vi "Read configuration.vi"(7 "force loading?":bool=TRUE, 8 "error in (no error)":errorcluster, 11 "DAQMH121119OrcaFlash in":refnum<class "DAQOrcaFlash.lvclass">) -> (0 "error out":errorcluster, 3 "DAQMH121119OrcaFlash out":refnum<class "DAQOrcaFlash.lvclass">)   [LabVIEW 2012, in "DAQOrcaFlash.lvclass"]
doc: "Reads the XML-based configuration file and populates the configuration cluster accordingly. Configuration file name is <component ID>.xml."
uses:
  DAQOrcaFlash.lvclass
  <vilib>/Distrio/Murmex/Murmex/Murmex.lvclass
  DAQOrcaFlash.lvclass/DAQOrcaFlash.ctl
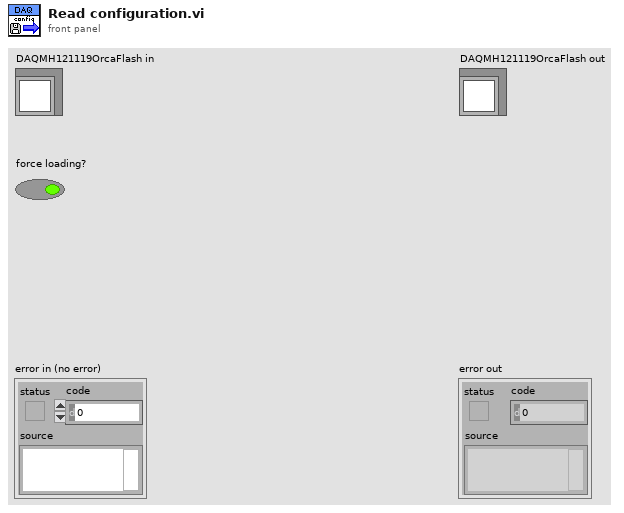
[diagram p1: front panel]
types:
  T1 = typedef "DAQOrcaFlash.lvclass/configuration_cluster.ctl" = cluster{"filepath":path, "Trigger source":T2, "Trigger mode":T3, "Sensor mode":T4, "Read out direction":T5, "Output trigger type":T6, "Output trigger source":T7, "Output trigger period":sgl[unit], "start_stop_targets":string[], "Output trigger connector":T8, "Stack component":string, "Tomo component":string, "auxiliary folder path":path, "wait before acquisition":dbl[unit], "maximum window size":i32}
  T2 = typedef "DAQOrcaFlash.lvclass/trigger_source.ctl" = sgl
  T3 = typedef "DAQOrcaFlash.lvclass/trigger_mode.ctl" = sgl
  T4 = typedef "DAQOrcaFlash.lvclass/sensor_mode.ctl" = sgl
  T5 = typedef "DAQOrcaFlash.lvclass/read out direction.ctl" = sgl
  T6 = typedef "DAQOrcaFlash.lvclass/output trigger type.ctl" = sgl
  T7 = typedef "DAQOrcaFlash.lvclass/output trigger source.ctl" = sgl
  T8 = typedef "DAQOrcaFlash.lvclass/connector.ctl" = enum32{"1", "2", "3"}
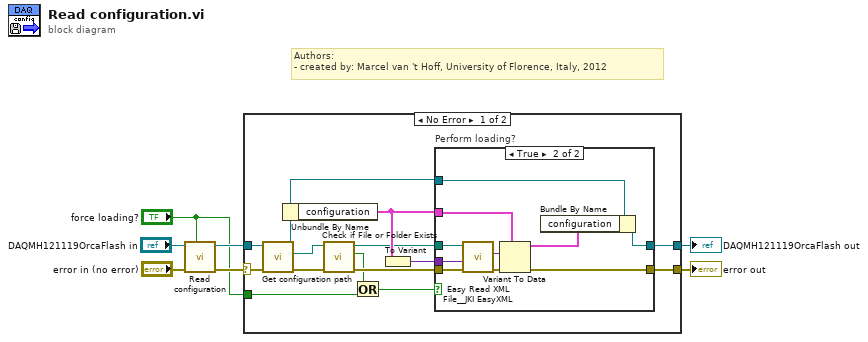
[diagram p0: block diagram]
diagram:
  # "Authors: \n- created by: Marcel van 't Hoff, University of Florence, Italy, 2012"
  n1 = call-parent "Read configuration.vi"("force loading?"="force loading?", "error in (no error)"="error in (no error)", "Murmex in"="DAQMH121119OrcaFlash in") -> ("error out"=w4:errorcluster, "Murmex out"=w5:refnum<class "DAQOrcaFlash.lvclass">)  [unwired: 7 in]
  n2 = case shown="No Error" w4 {
    selector: w4 -> [w10 w35]
    tunnel: [w18 w35] -> w1
    tunnel: [w21 w34] -> w2
    tunnel: w5 -> [w8 w34]
    tunnel: "force loading?" -> [w17 _]
    frame No Error {
      n3 = call <vilib>:"Get configuration path.vi"("error in (no error)"=w10, "Murmex in"=w8) -> ("error out"=w13:errorcluster, "configuration path"=w15:path, "Murmex out"=w9:refnum<class "DAQOrcaFlash.lvclass">)  [unwired: 7 in]
      n4 = Unbundle By Name(w9) -> ("configuration"=w19:T1)
      n5 = call <vilib>:"Check if File or Folder Exists.vi"("error in (no error)"=w13, "path"=w15) -> ("error out"=w12:errorcluster, "file or folder exists?"=w11:bool, "dup path"=w14:path)  [unwired: 7 in]
      n6 = Or(x=w11, y=w17) -> (x .or. y?=w16:bool)
      n7 = To Variant(anything=w19) -> (Variant=w20:variant)
      n8 = case "Perform loading?" shown="True" w16 {
        tunnel: [w23 w25] -> w21
        tunnel: w20 -> [_ w32]
        tunnel: w19 -> [_ w31]
        tunnel: [w22 w24] -> w18
        tunnel: w14 -> [_ w29]
        tunnel: w12 -> [w22 w28]
        tunnel: w9 -> [w23 w27]
        frame False {
        }
        frame True {
          n9 = call <vilib>:"Easy Read XML File__JKI EasyXML.vi"("error in (no error)"=w28, "LabVIEW Data (Type)"=w32, "XML File Path"=w29) -> ("error out"=w30:errorcluster, "LabVIEW Data"=w33:variant)  [unwired: 6 in, 1 out]
          n10 = Variant To Data(error in=w30, type=w31, Variant=w33) -> (data=w26:T1, error out=w24:errorcluster)
          n11 = Bundle By Name(cluster=w27, "configuration"=w26) -> (w25:refnum<class "DAQOrcaFlash.lvclass">)
        }
      }
    }
    frame Error {
    }
  }
  "error out" <- w1
  "DAQMH121119OrcaFlash out" <- w2
